vi "Check Record.vi"(8 "error in (no error)":errorcluster, 9 "Pulse file name":path=path "C:/Data", 10 "Log file name":path=path "C:/Data", 11 "Strain Logger in":refnum<class "Strain Logger.lvclass">) -> (0 "error out":errorcluster, 1 "Record exists":bool, 2 "tdms file out":refnum<k34>, 3 "Strain Logger out":refnum<class "Strain Logger.lvclass">)   [LabVIEW 2024, in "Strain Logger.lvclass"]
uses:
  Strain Logger.lvclass
  <vilib>/Utility/error.llb/Error Cluster From Error Code.vi
  <vilib>/ErrorRing/Error Ring.xnode
  Strain Logger.lvclass/Strain Logger.ctl
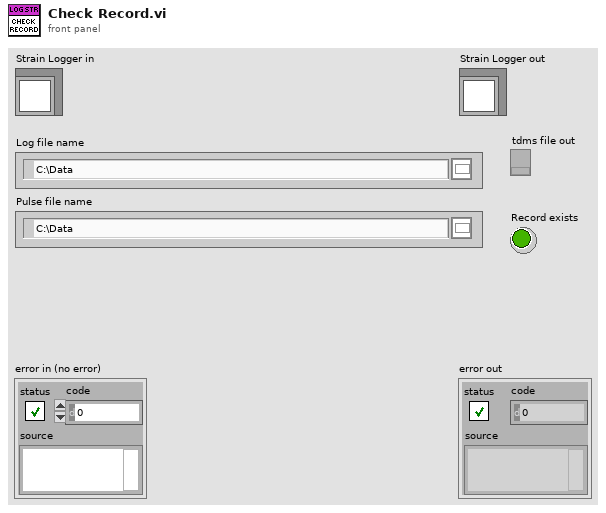
[diagram p1: front panel]
types:
  T1 = enum16{"open", "open or create", "create or replace", "create", "open (read-only)"}
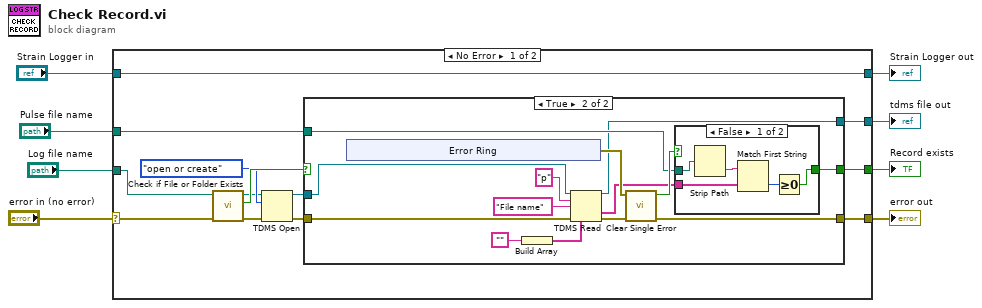
[diagram p0: block diagram]
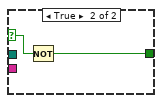
[diagram p3: hidden frame]
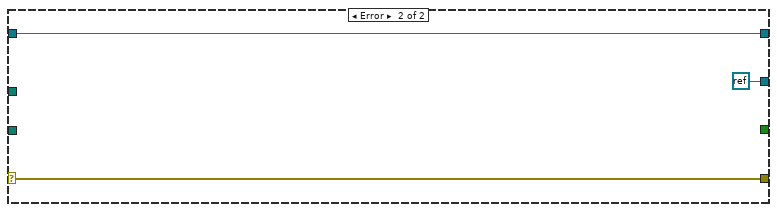
[diagram p4: hidden frame]
diagram:
  n1 = case shown="No Error" "error in (no error)" {
    selector: "error in (no error)" -> [w15 w52]
    tunnel: [w14 w52] -> w7
    tunnel: [w21 w51] -> w5
    tunnel: "Strain Logger in" -> [w21 w51]
    tunnel: "Log file name" -> [w20 _]
    tunnel: [w18 _] -> w3
    tunnel: "Pulse file name" -> [w16 _]
    tunnel: [w13 refnum<k0> refnum] -> w1
    frame No Error {
      n2 = call <vilib>:"Check if File or Folder Exists.vi"("error in (no error)"=w15, "path"=w20) -> ("error out"=w17:errorcluster, "file or folder exists?"=w19:bool, "dup path"=w11:path)  [unwired: 7 in]
      n3 = TDMS Open(8:w17, 10:T1."open or create" ("operation (0:open)"), 11:w11) -> (0:w10:errorcluster, 3:w9:refnum<k34>)  [unwired: 4 in]
      n4 = case shown="True" w19 {
        selector: w19 -> [w24 _]
        tunnel: [w24 w32] -> w18
        tunnel: w16 -> [_ w30]
        tunnel: [w23 w29] -> w14
        tunnel: [w22 w28] -> w13
        tunnel: w10 -> [w23 w27]
        tunnel: w9 -> [w22 w26]
        frame False {
        }
        frame True {
          n5 = xnode "Error Ring"() -> ("error out"=w34:errorcluster)
          n6 = Build Array("") -> (w31:string[])
          n7 = TDMS Read(0:w26, 5:"p" ("group name in"), 7:"File name" ("channel name(s) in"), 11:w27, 12:w31) -> (4:w28:refnum<k34>, 10:w25:string[], 15:w35:errorcluster)  [unwired: 3 in, 3 out]
          n8 = call "Clear Single Error.vi"("Error In"=w35, "Error to clear"=w34) -> ("Error Out"=w29:errorcluster, "specific error cleared?"=w33:bool)  [unwired: 8 in]
          n9 = case shown="False" w33 {
            selector: w33 -> [_ w45]
            tunnel: [w40 w44] -> w32
            tunnel: w25 -> [w43 _]
            tunnel: w30 -> [w42 _]
            frame False {
              n10 = Strip Path(path=w42) -> (name=w39:string)  [unwired: 1 out]
              n11 = Match First String(2:w43, 3:w39) -> (0:w41:i32)  [unwired: 1 out]
              n12 = Greater Or Equal To 0?(x=w41) -> (x >= 0?=w40:bool)
            }
            frame True {
              n13 = Not(x=w45) -> (.not. x?=w44:bool)
            }
          }
        }
      }
    }
    frame Error {
    }
  }
  "error out" <- w7
  "Strain Logger out" <- w5
  "Record exists" <- w3
  "tdms file out" <- w1
